vi "Configure Aurora Link.vi"(0 "niUsrpRio Session":T2={"FPGA Interface"=refnum, "RIO Interface Number"=0, "Data Clock Rate"=0, "FPGA Data Clock Rate"=0, "Global Settings Register Bus"=refnum, "Radio 0 Settings Register Bus"=refnum, "Radio 1 Settings Register Bus"=refnum, "Radio Settings Bus Semaphore"=refnum, "DB Queues"=[], "Characterization Data Valid?"=FALSE, "EEPROM Header"={"Checksum"=0, "Product Code"=0, "Hardware Current Version"=0, "Hardware Oldest Compatible Version"=0, "EEPROM Map Current Version"=0, "EEPROM Map Oldest Compatible Version"=0, "User Password"="", "Pointer to Factory Header"=0, "Pointer to User Header"=0, "Recommended Interval"=0, "Number of Reserved Bytes"=9, "Number of Daughterboards"=0, "Daughterboard IDs"=[], "Daughterboard Serial Numbers"=[]}, "Device Data Header"={"Checksum"=0, "Number of Channels"=0, "Number of Gain Settings"=[], "Pointer to Characterization Data"=[], "Number of Reserved Bytes"=27, "Number of Frequencies"=[]}, "EEPROM Characterization Header"={"Checksum"=0, "Date"=timestamp(0 s since 1904-01-01), "Temperature"=0.0, "Misc. Info"="", "Pointer to Device Data Header"=0, "Number of Reserved Bytes"=28}, "Characterization Data"=[], "FPGA Current Version"=0, "FPGA Oldest Compatible Version"=0, "Fixed Logic Current Version"=0, "Fixed Logic Oldest Compatible Version"=0, "FPGA Radio Settings Bus Current Version"=0, "FPGA Radio Settings Bus Oldest Compatible Version"=0, "FPGA Board Config Current Version"=0, "FPGA Board Config Oldest Compatible Version"=0, "Daughterboard Clock Rate"=0, "daughterboard configuration session handles"=[]} {"Daughterboard Clock Rate" format="%#.3pHz"; "FPGA Data Clock Rate" format="%#.3pHz"; "Data Clock Rate" format="%#.3pHz"; "Characterization Data"."Frequencies [Hz]" format="%#_6p"; "EEPROM Characterization Header"."Pointer to Device Data Header" format="%x"; "EEPROM Characterization Header"."Checksum" format="%x"; "Device Data Header"."Pointer to Characterization Data" format="%x"; "Device Data Header"."Checksum" format="%x"; "EEPROM Header"."Pointer to User Header" format="%x"; "EEPROM Header"."Pointer to Factory Header" format="%x"; "EEPROM Header"."Product Code" format="%x"; "EEPROM Header"."Checksum" format="%x"}, 5 "data stream config":enum16{"SFP Port 0", "SFP Port 1", "Host"}(ring)=enum."Host", 11 "error in":errorcluster) -> (4 "niUsrpRio Session (out)":T2 {"Daughterboard Clock Rate" format="%#.3pHz"; "FPGA Data Clock Rate" format="%#.3pHz"; "Data Clock Rate" format="%#.3pHz"; "Characterization Data"."Frequencies [Hz]" format="%#_6p"; "EEPROM Characterization Header"."Pointer to Device Data Header" format="%x"; "EEPROM Characterization Header"."Checksum" format="%x"; "Device Data Header"."Pointer to Characterization Data" format="%x"; "Device Data Header"."Checksum" format="%x"; "EEPROM Header"."Pointer to User Header" format="%x"; "EEPROM Header"."Pointer to Factory Header" format="%x"; "EEPROM Header"."Product Code" format="%x"; "EEPROM Header"."Checksum" format="%x"}, 6 "Ports debug":T1(array[cluster]), 15 "error out":errorcluster)   [LabVIEW 2016]
uses:
  <instrlib>/niUsrpRio/Config/v1/Host/Public/niUsrpRio Session.ctl
  <instrlib>/_niInstr/Register Bus/v0/Host/Public/Register Bus Session.ctl
  <instrlib>/_niInstr/Register Bus/v0/Host/Private/Session Data.ctl
  <instrlib>/niUsrpRio/Config/v1/Host/Private/DB Queue Reference.ctl
  <instrlib>/niUsrpRio/Config/v1/Host/Private/Daughterboard Data.ctl
  <instrlib>/niUsrpRio/Config/v1/Host/Private/ATR state data.ctl
  <instrlib>/niUsrpRio/Config/v1/Host/Private/Antenna Configuration.ctl
  <instrlib>/niUsrpRio/Config/v1/Host/Private/CPLD Power Mode.ctl
  <instrlib>/niUsrpRio/Config/v1/Host/Public/EEPROM Header.ctl
  <instrlib>/niUsrpRio/Config/v1/Host/Public/EEPROM Device Data Header.ctl
  <instrlib>/niUsrpRio/Config/v1/Host/Public/EEPROM Characterization Header.ctl
  <instrlib>/niUsrpRio/Config/v1/Host/Public/Characterization Data.ctl
  <instrlib>/niUsrpRio/Config/v1/Host/Public/IQ Imbalance.ctl
  Aurora FPGA Ref.ctl
  Port.ctl
  <vilib>/rvi/errors/niLvFpgaAdjustHostInterfaceError.vi
  <vilib>/Utility/error.llb/Error Cluster From Error Code.vi
  <vilib>/rvi/interface/nirviReadWriteControl/nirviReadWriteControl.xnode
  <vilib>/rvi/interface/Simulation/niFpgaSimulationCallBeginRW.vi
  NiFpgaLv.dll
  <instrlib>/niUsrpRio/Config/v1/Host/niUsrpRio Config v1 Host.lvlib
  <instrlib>/_niInstr/Register Bus/v0/Host/niInstr Register Bus v0 Host.lvlib
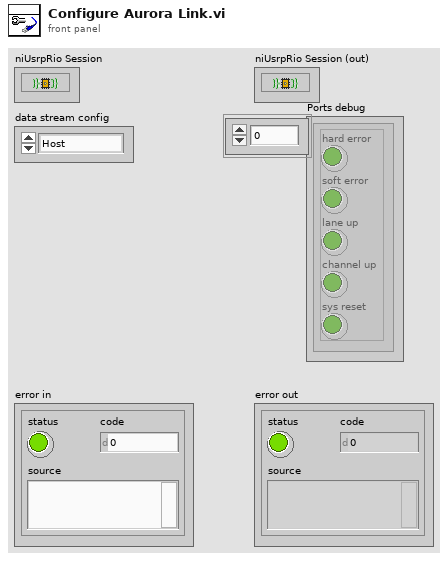
[diagram p1: front panel]
types:
  T1 = cluster{"hard error":bool, "soft error":bool, "lane up":bool, "channel up":bool, "sys reset":bool}[]
  T2 = typedef "niUsrpRio Config v1 Host.lvlib/niUsrpRio Session.ctl" = cluster{"FPGA Interface":refnum<k20>, "RIO Interface Number":u32, "Data Clock Rate":u32, "FPGA Data Clock Rate":u32, "Global Settings Register Bus":T3, "Radio 0 Settings Register Bus":T3, "Radio 1 Settings Register Bus":T3, "Radio Settings Bus Semaphore":T4, "DB Queues":T5[], "Characterization Data Valid?":bool, "EEPROM Header":T6, "Device Data Header":T7, "EEPROM Characterization Header":T8, "Characterization Data":T9[], "FPGA Current Version":u32, "FPGA Oldest Compatible Version":u32, "Fixed Logic Current Version":u32, "Fixed Logic Oldest Compatible Version":u32, "FPGA Radio Settings Bus Current Version":u32, "FPGA Radio Settings Bus Oldest Compatible Version":u32, "FPGA Board Config Current Version":u32, "FPGA Board Config Oldest Compatible Version":u32, "Daughterboard Clock Rate":u32, "daughterboard configuration session handles":u64[]}
  T3 = typedef "niInstr Register Bus v0 Host.lvlib/Register Bus Session.ctl" = refnum<queue>
  T4 = typedef "Semaphore RefNum" = refnum<k1>
  T5 = typedef "niUsrpRio Config v1 Host.lvlib/DB Queue Reference.ctl" = refnum<queue>
  T6 = typedef "niUsrpRio Config v1 Host.lvlib/EEPROM Header.ctl" = cluster{"Checksum":u32, "Product Code":u16, "Hardware Current Version":u16, "Hardware Oldest Compatible Version":u16, "EEPROM Map Current Version":u16, "EEPROM Map Oldest Compatible Version":u16, "User Password":string, "Pointer to Factory Header":u32, "Pointer to User Header":u32, "Recommended Interval":u16, "Number of Reserved Bytes":i32, "Number of Daughterboards":u8, "Daughterboard IDs":u16[], "Daughterboard Serial Numbers":string[]}
  T7 = typedef "niUsrpRio Config v1 Host.lvlib/EEPROM Device Data Header.ctl" = cluster{"Checksum":u32, "Number of Channels":u8, "Number of Gain Settings":u16[], "Pointer to Characterization Data":u32[], "Number of Reserved Bytes":i32, "Number of Frequencies":u16[]}
  T8 = typedef "niUsrpRio Config v1 Host.lvlib/EEPROM Characterization Header.ctl" = cluster{"Checksum":u32, "Date":timestamp, "Temperature":sgl, "Misc. Info":string, "Pointer to Device Data Header":u32, "Number of Reserved Bytes":i32}
  T9 = typedef "niUsrpRio Config v1 Host.lvlib/Characterization Data.ctl" = cluster{"Gains[dB]":dbl[], "Frequencies [Hz]":dbl[], "IQ Imbalance Table":T10[], "Measured Gains[dB]":dbl[][]}
  T10 = typedef "niUsrpRio Config v1 Host.lvlib/IQ Imbalance.ctl" = cluster{"Gain Imbalance [linear]":dbl, "Phase Imbalance [radians]":dbl, "Offset":cdb}
  T11 = typedef "Aurora FPGA Ref.ctl" = refnum<k20>
  T12 = typedef "niUsrpRio Config v1 Host.lvlib/DB Types.ctl" = enum16{"sbx", "cbx", "wbx", "unknown", "ubx", "twinrx"}
  T13 = typedef "Port.ctl" = i32
  T14 = cluster{"hard error":bool, "soft error":bool, "lane up":bool, "channel up":bool, "sys reset":bool}
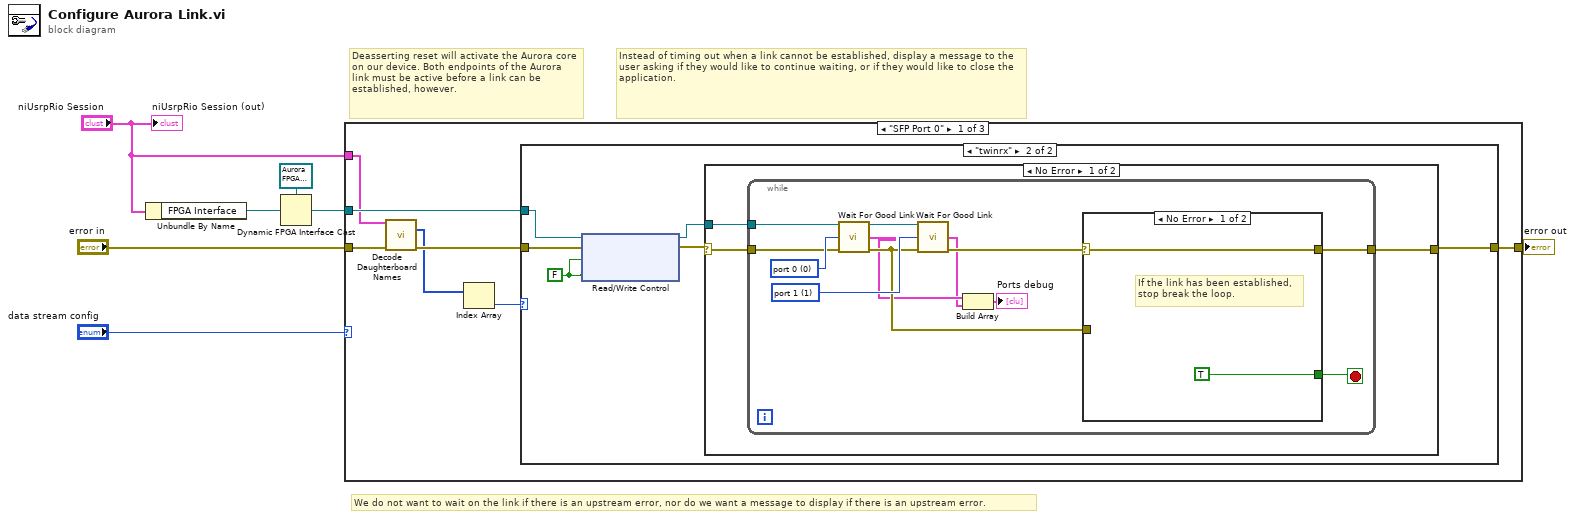
[diagram p0: block diagram]
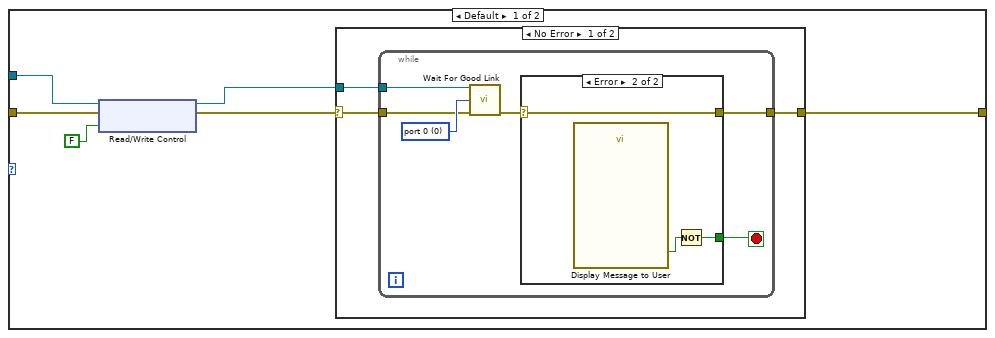
[diagram p2: hidden frame]
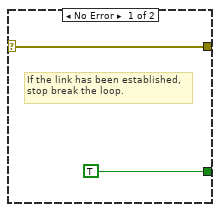
[diagram p3: hidden frame]
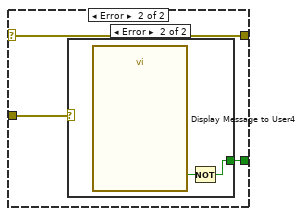
[diagram p5: hidden frame]
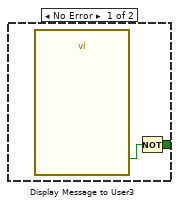
[diagram p6: hidden frame]
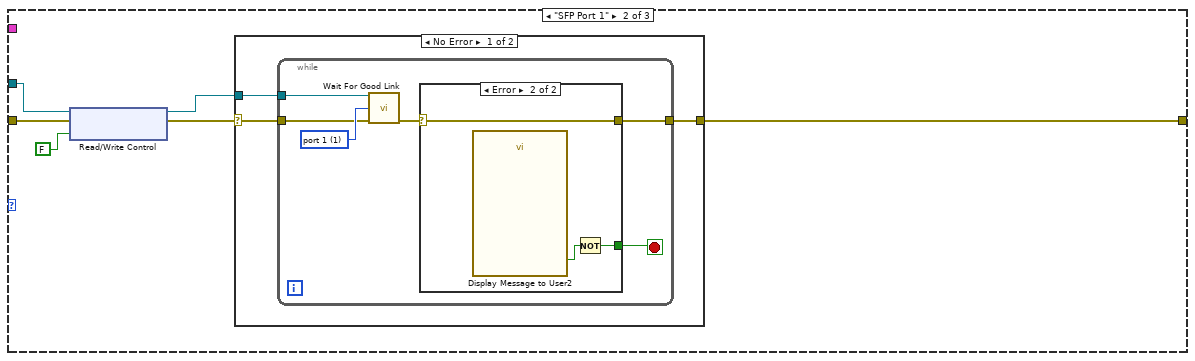
[diagram p8: hidden frame]
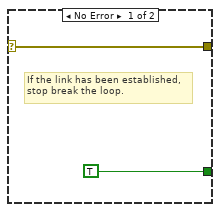
[diagram p9: hidden frame]
diagram:
  # "We do not want to wait on the link if there is an upstream error, nor do we want a message to display if there is an upstream error."
  # "Instead of timing out when a link cannot be established, display a message to the user asking if they would like to continue waiting, or if they would like to close the application."
  # "Deasserting reset will activate the Aurora core on our device. Both endpoints of the Aurora link must be active before a link can be established, however."
  n1 = Unbundle By Name("niUsrpRio Session") -> ("FPGA Interface"=w7:refnum<k20>)
  n2 = Dynamic FPGA Interface Cast(Session In=T11 refnum ("USRP RIO Streaming Xcvr FPGA VI Reference"), Type=w7) -> (Session Out=w6:T11)
  n3 = case shown="\"SFP Port 0\"" "data stream config" {
    tunnel: w6 -> [w14 w72 _]
    tunnel: "error in" -> [w12 w69 w88]
    tunnel: [w13 w67 w88] -> w3
    tunnel: "niUsrpRio Session" -> [w10 _ _]
    frame "SFP Port 0" {
      n4 = call <instrlib>:"Decode Daughterboard Names.vi"("niUsrpRio Session"=w10, "error in"=w12) -> ("daughterboard names"=w9:T12[], "error out"=w11:errorcluster)  [unwired: 11 in, 1 out]
      n5 = Index Array(array=w9) -> (element=w8:T12)  [unwired: 1 in]
      n6 = case shown="\"twinrx\"" w8 {
        tunnel: w14 -> [w20 w40]
        tunnel: [w16 w36] -> w13
        tunnel: w11 -> [w15 w41]
        frame Default {
          n7 = xnode "Read/Write Control"("FPGA VI Reference In"=w20, "error in"=w15, "sfp 0.core reset"=FALSE) -> ("FPGA VI Reference Out"=w19:T11, "error out"=w17:errorcluster)
          n8 = case shown="No Error" w17 {
            selector: w17 -> [w22 w35]
            tunnel: w19 -> [w23 _]
            tunnel: [w21 w35] -> w16
            frame No Error {
              n9 = while {
                tunnel: w23 -> [w26]
                tunnel: [w25] -> w21
                tunnel: w22 -> [w24]
                stop <- w27 stop-if-true
                w29 = T13 0 items=["port 0", "port 1"] ("Port")
                n10 = call "Wait For Good Link.vi"("refnum in"=w26, "port"=w29, "error in"=w24) -> ("error out"=w28:errorcluster)  [unwired: 10 in, 2 out]
                n11 = case shown="Error" w28 {
                  selector: w28 -> [w30 w32]
                  tunnel: [TRUE w34] -> w27
                  tunnel: [w30 w32] -> w25
                  frame No Error {
                    # "If the link has been established,\nstop break the loop."
                  }
                  frame Error {
                    n12 = call "Display Message to User"() -> ("OK"=w33:bool)  [unwired: 10 in, 1 out]
                    n13 = Not(x=w33) -> (.not. x?=w34:bool)
                  }
                }
              }
            }
            frame Error {
            }
          }
        }
        frame "twinrx" {
          w39 = FALSE
          n14 = xnode "Read/Write Control"("FPGA VI Reference In"=w40, "error in"=w41, "sfp 0.core reset"=w39, "sfp 1.core reset"=w39) -> ("FPGA VI Reference Out"=w37:T11, "error out"=w38:errorcluster)
          n15 = case shown="No Error" w38 {
            selector: w38 -> [w43 w66]
            tunnel: w37 -> [w44 _]
            tunnel: [w42 w66] -> w36
            frame No Error {
              n16 = while {
                tunnel: w44 -> [w54]
                tunnel: [w49] -> w42
                tunnel: w43 -> [w53]
                stop <- w55 stop-if-true
                w51 = T13 1 items=["port 0", "port 1"] ("port")
                w56 = T13 0 items=["port 0", "port 1"] ("Port")
                n17 = call "Wait For Good Link.vi"("refnum in"=w54, "port"=w56, "error in"=w53) -> ("refnum out"=w52:T11, "port debug info"=w47:T14, "error out"=w48:errorcluster)  [unwired: 10 in]
                n18 = call "Wait For Good Link.vi"("refnum in"=w52, "port"=w51, "error in"=w48) -> ("port debug info"=w46:T14, "error out"=w50:errorcluster)  [unwired: 10 in, 1 out]
                n19 = Build Array(w47, w46) -> (→"Ports debug":T1)
                n20 = case shown="No Error" w50 {
                  selector: w50 -> [w57 w60]
                  tunnel: [TRUE w61] -> w55
                  tunnel: [w57 w60] -> w49
                  tunnel: w48 -> [_ w59]
                  frame No Error {
                    # "If the link has been established,\nstop break the loop."
                  }
                  frame Error {
                    n21 = case shown="Error" w59 {
                      tunnel: [w63 w64] -> w61
                      frame No Error {
                        n22 = call "Display Message to User3"() -> ("OK"=w62:bool)  [unwired: 10 in, 1 out]
                        n23 = Not(x=w62) -> (.not. x?=w63:bool)
                      }
                      frame Error {
                        n24 = call "Display Message to User4"() -> ("OK"=w65:bool)  [unwired: 10 in, 1 out]
                        n25 = Not(x=w65) -> (.not. x?=w64:bool)
                      }
                    }
                  }
                }
              }
            }
            frame Error {
            }
          }
        }
      }
    }
    frame "SFP Port 1" {
      n26 = xnode "Read/Write Control"("FPGA VI Reference In"=w72, "error in"=w69, "sfp 1.core reset"=FALSE) -> ("FPGA VI Reference Out"=w71:T11, "error out"=w68:errorcluster)
      n27 = case shown="No Error" w68 {
        selector: w68 -> [w74 w87]
        tunnel: w71 -> [w75 _]
        tunnel: [w73 w87] -> w67
        frame No Error {
          n28 = while {
            tunnel: w75 -> [w78]
            tunnel: [w77] -> w73
            tunnel: w74 -> [w76]
            stop <- w79 stop-if-true
            w81 = T13 1 items=["port 0", "port 1"] ("Port")
            n29 = call "Wait For Good Link.vi"("refnum in"=w78, "port"=w81, "error in"=w76) -> ("error out"=w80:errorcluster)  [unwired: 10 in, 2 out]
            n30 = case shown="Error" w80 {
              selector: w80 -> [w82 w84]
              tunnel: [TRUE w86] -> w79
              tunnel: [w82 w84] -> w77
              frame No Error {
                # "If the link has been established,\nstop break the loop."
              }
              frame Error {
                n31 = call "Display Message to User2"() -> ("OK"=w85:bool)  [unwired: 10 in, 1 out]
                n32 = Not(x=w85) -> (.not. x?=w86:bool)
              }
            }
          }
        }
        frame Error {
        }
      }
    }
    frame Default {
    }
  }
  "error out" <- w3
  "niUsrpRio Session (out)" <- "niUsrpRio Session"
